vi "Create_Trajectory_Using_PathfinderSwerve_ORIG.vi"() -> ()   [LabVIEW 2019]
uses:
  <vilib>/Rock Robotics/WPI/ThirdParty/JAS_Junk/JaciPathFinderLib/VIs/Waypoint.ctl
  <vilib>/Rock Robotics/WPI/ThirdParty/JAS_Junk/TrajLib/TRAJ_STATE.ctl
  <vilib>/Rock Robotics/WPI/ThirdParty/JAS_Junk/TrajLib/POSE2D.ctl
  <vilib>/Rock Robotics/WPI/ThirdParty/JAS_Junk/TrajLib/TRANSLATION2D.ctl
  <vilib>/Rock Robotics/WPI/ThirdParty/JAS_Junk/TrajLib/ROTATION2D.ctl
  <vilib>/Rock Robotics/WPI/ThirdParty/JAS_Junk/TrajLib/UTIL_PATHFINDER_CONFIG.ctl
  <vilib>/Rock Robotics/WPI/ThirdParty/JAS_Junk/TrajLib/DISPLAY_WAYPOINT.ctl
  <vilib>/Rock Robotics/WPI/ThirdParty/JAS_Junk/JaciPathFinderLib/Pathfinder.lvlib
  <vilib>/Rock Robotics/WPI/ThirdParty/JAS_Junk/TrajLib/Trajectory_Library.lvlib
panel:
  in  "End Program":bool
  in  "Tab Control":T1(tab)
  in  "max_velocity":dbl=58.0
  in  "max_acceleration":dbl=65.0
  in  "max_jerk":dbl=70.0
  in  "wheelbase_width":dbl=20.866
  in  "Real max\n speed":dbl=65.0
  in  "wheelbase_depth":dbl=28.0
  in  "mode":u32(ring) items=["SWERVE_DEFAULT"]
  out "max speed":dbl
  out "Path \nSpeed > \nMax":bool
  out "Complete,\nReady to \nSave file":bool
  in  "Calculate\nPath":bool
  out "Path calculation error":errorcluster
  in  "sample_count":i32=100000
  in  "Path Results\ndT":dbl=0.02 format="%7.3f"
  in  "?":T2[](array[typedef])=[{"x"=15.0, "y"=105.0, "angle"=-45.0}, {"x"=105.0, "y"=65.0, "angle"=0.0}, {"x"=210.0, "y"=106.0, "angle"=45.0}]
  out "Position":cluster{dbl[], dbl[]}[](graph)
  out "Path Data":cluster{dbl[], dbl[]}[](graph)
  out "Traj States\nSize":i32
  out "Trajectory States":T3[](array[typedef]) {"POSE"."ROTATION"."SIN" format="%13.4f"; "POSE"."ROTATION"."COS" format="%13.4f"; "POSE"."ROTATION"."VALUE" format="%13.4f"; "POSE"."TRANSLATION"."Y" format="%14.3f"; "POSE"."TRANSLATION"."X" format="%14.3f"}
  out "File Saved\nWithout\nError":bool
  in  "Trajectory Type":enum32{"Radio Selection 1", "Radio Selection 2"}(radio)
  out "File Creation\nError":errorcluster
  in  "Trajectory File Comment":string
  in  "Trajectory File Name":path
  in  "CreateCmdList":bool
  # "Create trajectory using \"Jaci's Pathfinder\"  (Display for swerve drive robot)"
  # "Instructions:\n----------------  \nThis utility will create a trajectory,, show the data on the various tabs, and optionally write a \"robot relative\" trajectory to a \nfile. To use this utility:\n\n1) Read all of these instructions!\n2) Define the Robot Data. on the \"Robot Data\" tab.\n3) Define the \"Path Definition\" on the \"Define / Create Trajectory\" tab.  These are the beginning and ending positions/headings, and \n     internal positions/headings.\n4) Define the time increment.  0.020 is chosen since that matches the normal robot loop time.\n5) Define \"sample count\".  This is an internal PathFinder variable.  Leaving the value as default should work correctly.  Making \n    the value a little smaller will speed the program up a little.\n6) Press the \"Calculate Path\".  If a good path was calculated it will be displayed on the \"Field Position tab, and the \"Complete, \n    Ready to Save\" indicator will light.  The path can be recalculated many times before performing any other action.\n\nAfter a Path has been calculated, the \"trajectory can be written to a file.  The absolute path is converted to a robot relative \ntrajectory.  To do this:\n1) Enter a comment to be included in the file.  Anything can be entered.\n2) Select the file name.\n3) Select the type of trajectory to save, absolute or relative.\n4) Press \"Create Trajectory File\"  If an error occurs it will be displayed in the File Creation Error indicator.\n\nNotes:\n---------\n- All the robot parameters, path, and field dimensions are in INCHES, and DEGREES.  The resulting trajectory is converted to \n   METERS, and RADIANS to match the rest of this library!\n- The pathfinder path generation logic doesn't account distribution of speed to the left and right wheels.  As a result the \n   maximum speed can be exceeded.If this happens, but Path Speed > Max light will light and Ready to Execute will not \n   light.  Lower the maximum speed in the Robot Data tab and recalulate the path.  (CURRENTLY THIS LOGIC IS NOT COMPLETE.)\n- 2019 playing field size - width: 26 ft 11.25 In = 323.25 in , length: 52 ft 5.25 in = 629.25 in  (I didn't verify this for the 2020 version.)"
  # "ROBOT DATA"
  # "INCHES/SEC"
  # "INCHES/SEC"
  # "INCHES/SEC^2"
  # "INCHES/SEC^3"
  # "Simulated robot wheelbase is: 20.866"
  # "INCHES"
  # "Simulated robot max speed is: 68.266"
  # "INCHES"
  # "PATH DEFINITION"
  # "SEC"
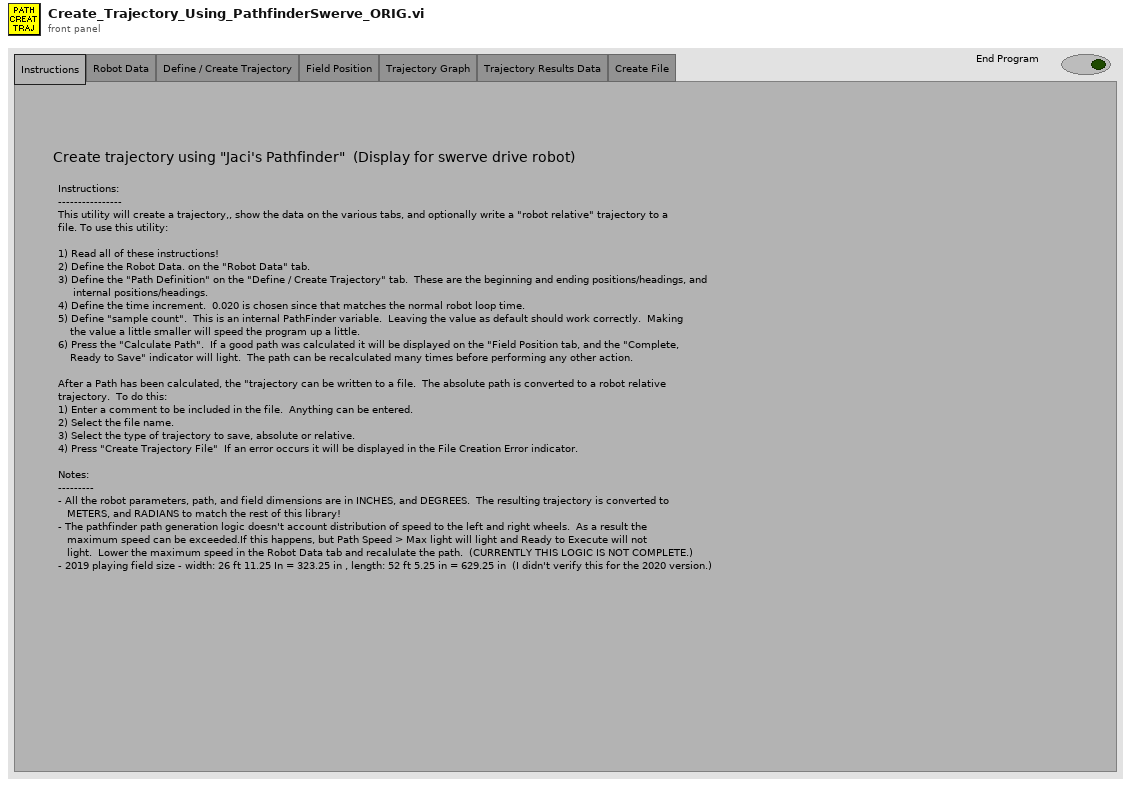
[diagram p1: front panel]
types:
  T1 = enum32{"Instructions", "Robot Data", "Define / Create Trajectory", "Field Position", "Trajectory Graph", "Trajectory Results Data", "Create File"}
  T2 = typedef "Pathfinder.lvlib/Waypoint.ctl" = cluster{"x":dbl, "y":dbl, "angle":dbl}
  T3 = typedef "Trajectory_Library.lvlib/TRAJ_STATE.ctl" = cluster{"TimeSeconds":dbl, "Velocity":dbl, "Acceleration":dbl, "POSE":T4, "Curvature":dbl}
  T4 = typedef "Trajectory_Library.lvlib/POSE2D.ctl" = cluster{"TRANSLATION":T5, "ROTATION":T6}
  T5 = typedef "Trajectory_Library.lvlib/TRANSLATION2D.ctl" = cluster{"X":dbl, "Y":dbl}
  T6 = typedef "Trajectory_Library.lvlib/ROTATION2D.ctl" = cluster{"VALUE":dbl, "COS":dbl, "SIN":dbl}
  T7 = typedef "Trajectory_Library.lvlib/DISPLAY_WAYPOINT.ctl" = cluster{"X":dbl, "Y":dbl, "ANGLE":dbl}
  T8 = typedef "Trajectory_Library.lvlib/UTIL_PATHFINDER_CONFIG.ctl" = cluster{"PathfinderType - 0 tank 1 serve":i32, "PathMaxVelocity - inches per sec":dbl, "MaxAcceleration - inches per sec2":dbl, "MaxJerk--Inches per sec2":dbl, "TimeDelta-Seconds":dbl, "SampleCount":i32, "WheelbaseWidth-inches":dbl, "WheelbaseDepth-inches":dbl, "SwerveType":i32, "ActualMaxVelocity-inches per sec":dbl}
  T9 = typedef "Trajectory_Library.lvlib/TRAJECTORY.ctl" = cluster{"TotalTImeSecs":dbl, "States":T3[]}
  T10 = typedef "Pathfinder.lvlib/Segment.ctl" = cluster{"dt":dbl, "x":dbl, "y":dbl, "position":dbl, "velocity":dbl, "acceleration":dbl, "jerk":dbl, "heading":dbl}
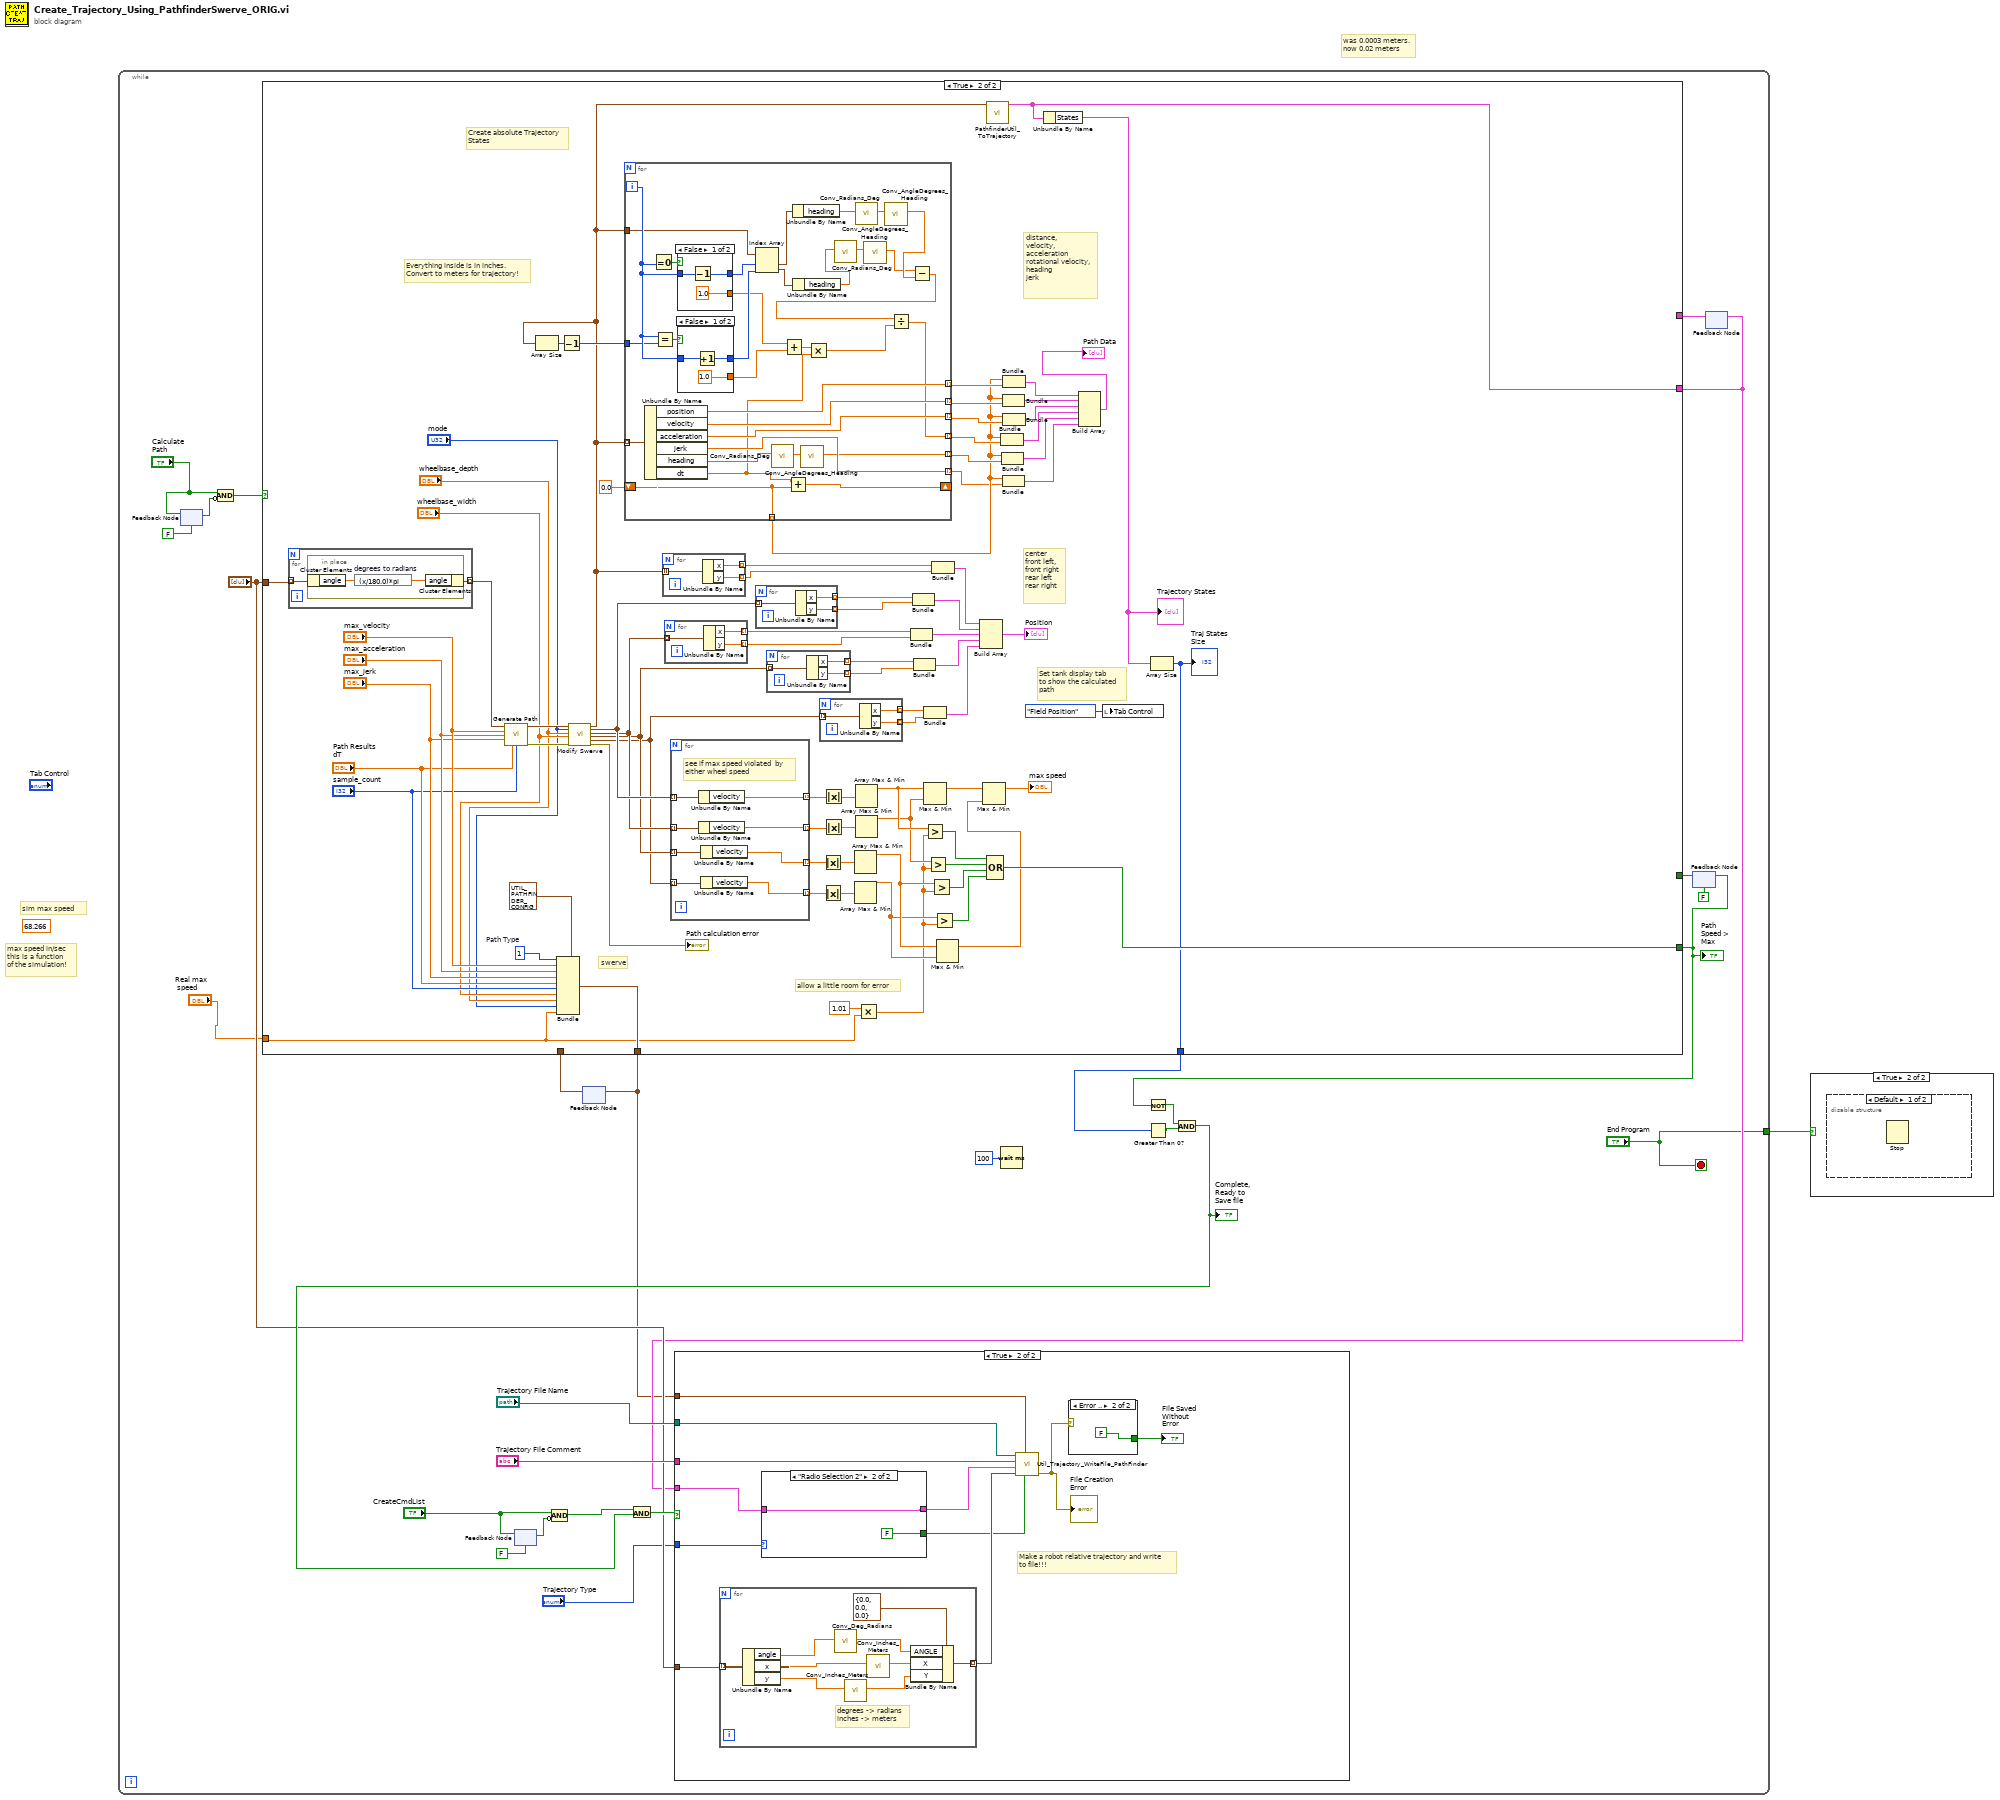
[diagram p0: block diagram]
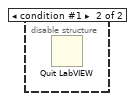
[diagram p3: hidden frame]
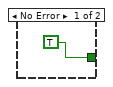
[diagram p5: hidden frame]
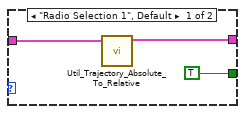
[diagram p6: hidden frame]
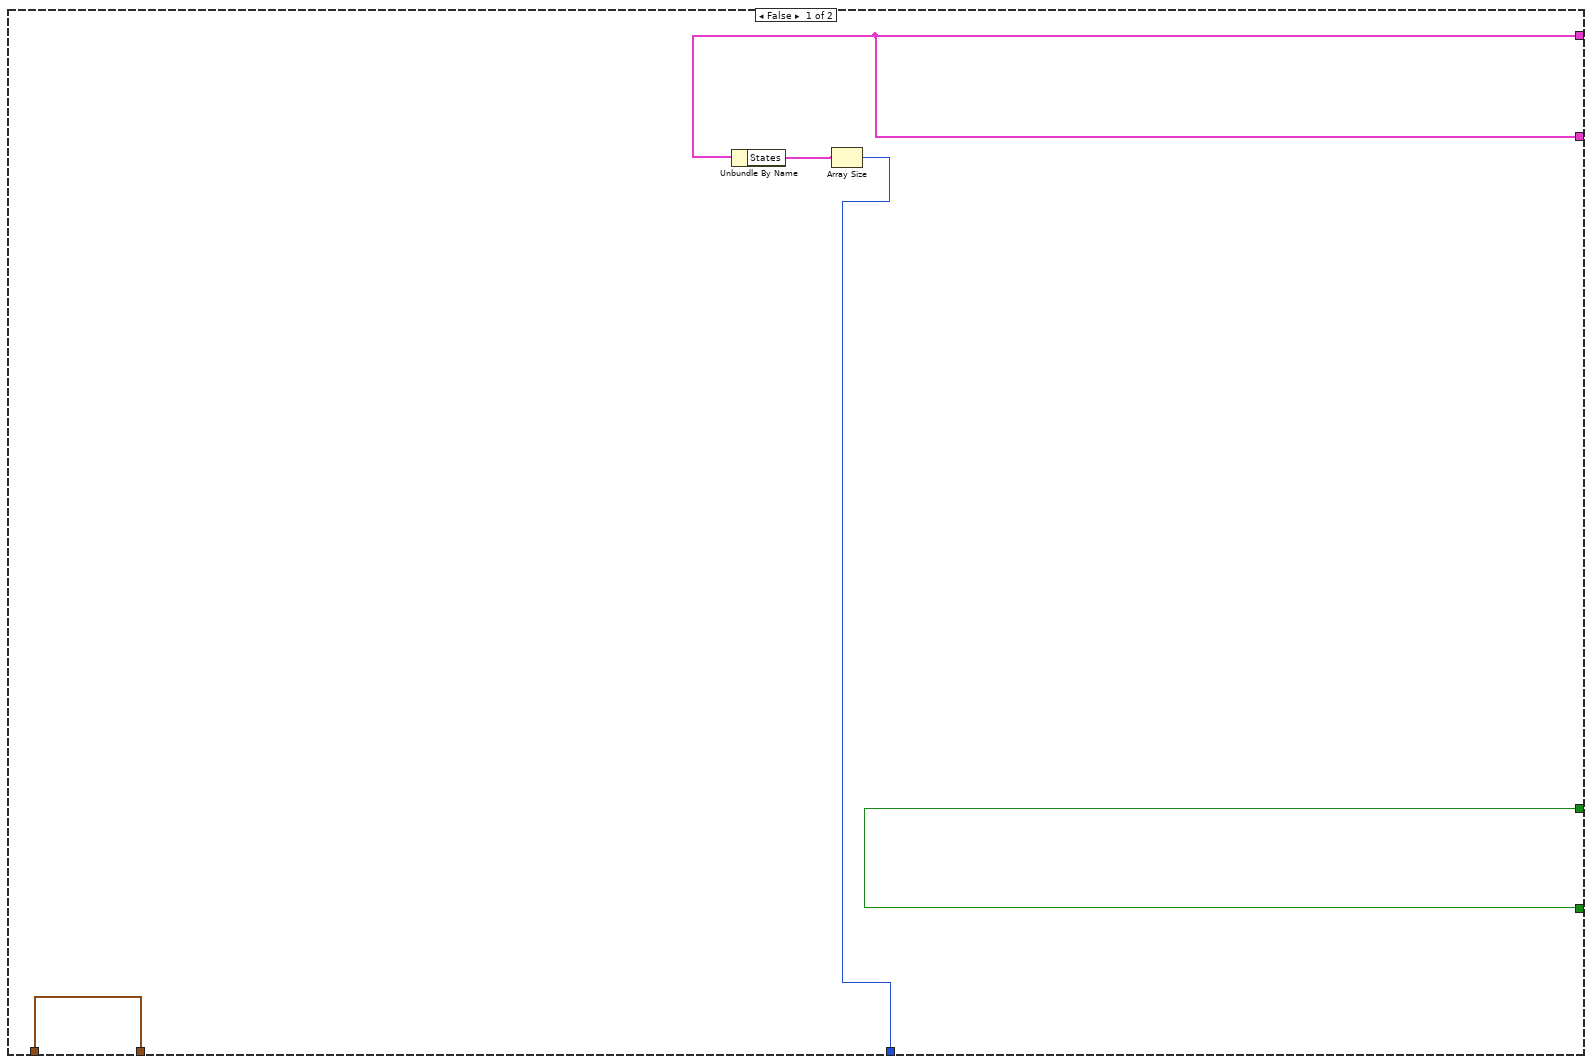
[diagram p7: hidden frame]
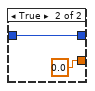
[diagram p8: hidden frame]
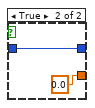
[diagram p9: hidden frame]
diagram:
  (unwired) 68.266 ("x")
  # "was 0.0003 meters.\nnow 0.02 meters"
  # "sim max speed"
  # "max speed in/sec\nthis is a function\nof the simulation!"
  n1 = while {
    tunnel: ["End Program"] -> w1
    stop <- "End Program" stop-if-true
    n2 = feedback #1(FALSE ("CreateCmdList")) -> (w10:bool)
    n3 = feedback-in #1("Calculate\nPath") -> ()
    n4 = Compound Arithmetic op=AND("Calculate\nPath", invert w10) -> (w7:bool)
    n5 = feedback-in #2("CreateCmdList") -> ()
    n6 = feedback #2(FALSE ("CreateCmdList")) -> (w13:bool)
    n7 = Compound Arithmetic op=AND("CreateCmdList", invert w13) -> (w12:bool)
    n8 = feedback #3() -> (w2:T8)  [unwired: 1 in]
    n9 = Wait (ms)(milliseconds to wait=u32 100) -> ()  [unwired: 1 out]
    n10 = feedback #4(FALSE) -> (w26:bool)
    n11 = feedback #5() -> (w22:T9)  [unwired: 1 in]
    n12 = case shown="True" w7 {
      tunnel: "Real max\n speed" -> [_ w62]
      tunnel: [w60 w127] -> w23
      tunnel: w26 -> [w60 _]
      tunnel: "?" -> [_ w126]
      tunnel: [w57 w106] -> w16
      tunnel: w22 -> [w57 _]
      tunnel: [w59 w120] -> w15
      tunnel: [w56 w65] -> w3
      tunnel: w2 -> [w56 _]
      frame False {
        n13 = Unbundle By Name(w57) -> ("States"=w58:T3[])
        n14 = Array Size(array=w58) -> (size(s)=w59:i32)
      }
      frame True {
        w74 = 1  # Path Type
        # "allow a little room for error"
        # "center\nfront left,\nfront right\nrear left\nrear right"
        # "distance,\nvelocity,\nacceleration\nrotational velocity,\nheading\njerk"
        # "swerve"
        # "Everything inside is in inches.\nConvert to meters for trajectory!"
        # "Create absolute Trajectory\nStates"
        # "Set tank display tab\nto show the calculated\npath"
        n15 = for {
          tunnel: w126 -> [w157] mode=indexing
          tunnel: [w156] -> w139 mode=indexing
          n16 = in-place {
            n17 = in-place-cluster #6(w157) -> ("angle"=w159:dbl)
            n18 = expression code="(x/180.0)*pi" "degrees to radians"(w159) -> (w158:dbl)
            n19 = in-place-cluster #6("angle"=w158) -> (w156:T2)
          }
        }
        n20 = call <vilib>:"Generate Path.vi"("path"=w139, "max_velocity"="max_velocity", "max_acceleration"="max_acceleration", "max_jerk"="max_jerk", "dt (.001)"="Path Results\ndT", "sample_count (100000)"="sample_count") -> ("Segments"=w140:T10[], "error out"=w96:errorcluster)  [unwired: 8 in]
        n21 = Bundle(cluster=T8 {"PathfinderType - 0 tank 1 serve"=0, "PathMaxVelocity - inches per sec"=0.0, "MaxAcceleration - inches per sec2"=0.0, "MaxJerk--Inches per sec2"=0.0, "TimeDelta-Seconds"=0.0, "SampleCount"=0, "WheelbaseWidth-inches"=0.0, "WheelbaseDepth-inches"=0.0, "SwerveType"=0, "ActualMaxVelocity-inches per sec"=0.0} ("UTIL_PATHFINDER_CONFIG"), "PathfinderType - 0 tank 1 serve"=w74, "PathMaxVelocity - inches per sec"="max_velocity", "MaxAcceleration - inches per sec2"="max_acceleration", "MaxJerk--Inches per sec2"="max_jerk", "TimeDelta-Seconds"="Path Results\ndT", "SampleCount"="sample_count", "WheelbaseWidth-inches"="wheelbase_width", "WheelbaseDepth-inches"="wheelbase_depth", "SwerveType"="mode", "ActualMaxVelocity-inches per sec"=w62) -> (w65:T8)
        n22 = call <vilib>:"Modify Swerve.vi"("Original"=w140, "mode"="mode", "wheelbase_depth"="wheelbase_depth", "wheelbase_width"="wheelbase_width", "error in"=w96) -> ("Original"=w97:T10[], "front_left out"=w80:T10[], "front_right out"=w79:T10[], "back_left out"=w78:T10[], "back_right out"=w77:T10[], "error out"=→"Path calculation error":errorcluster)  [unwired: 9 in]
        n23 = Array Size(array=w97) -> (size(s)=w99:i32)
        n24 = Decrement(x=w99) -> (x-1=w98:i32)
        n25 = for {
          tunnel: w97 -> [w200] mode=indexing
          shift-right: [w198] -> _
          shift-left: 0.0 -> [w199]
          tunnel: [w199] -> w102 mode=indexing
          tunnel: [w191] -> w103 mode=indexing
          tunnel: [w197] -> w101 mode=indexing
          tunnel: [w196] -> w111 mode=indexing
          tunnel: [w195] -> w110 mode=indexing
          tunnel: [w194] -> w105 mode=indexing
          tunnel: [w177] -> w104 mode=indexing
          tunnel: w97 -> [w183]
          tunnel: w98 -> [w176]
          i -> [w188]
          n26 = Unbundle By Name(w200) -> ("position"=w194:dbl, "velocity"=w195:dbl, "acceleration"=w196:dbl, "jerk"=w197:dbl, "heading"=w193:dbl, "dt"=w179:dbl)
          n27 = Equal To 0?(x=w188) -> (x = 0?=w190:bool)
          n28 = Equal?(x=w188, y=w176) -> (x = y?=w189:bool)
          n29 = case shown="False" w190 {
            tunnel: w188 -> [w208 w209]
            tunnel: [1.0 0.0] -> w180
            tunnel: [w206 w209] -> w185
            frame False {
              n30 = Decrement(x=w208) -> (x-1=w206:i32)
            }
            frame True {
            }
          }
          n31 = case shown="False" w189 {
            tunnel: [1.0 0.0] -> w181
            tunnel: w188 -> [w202 w204]
            tunnel: [w201 w204] -> w184
            frame False {
              n32 = Increment(x=w202) -> (x+1=w201:i32)
            }
            frame True {
            }
          }
          n33 = Index Array(array=w183, index #1=w185, index #2=w184) -> (element #1=w187:T10, element #2=w186:T10)
          n34 = call <vilib>:"Conv_Radians_Deg.vi"("Radians"=w193) -> ("Degrees"=w192:dbl)  [unwired: 10 in]
          n35 = Add(x=w180, y=w181) -> (x+y=w182:dbl)
          n36 = Add(x=w179, y=w199) -> (x+y=w198:dbl)
          n37 = Unbundle By Name(w187) -> ("heading"=w173:dbl)
          n38 = Unbundle By Name(w186) -> ("heading"=w171:dbl)
          n39 = call <vilib>:"Conv_AngleDegrees_Heading.vi"("Degrees"=w192) -> ("Heading Degrees"=w191:dbl)  [unwired: 10 in]
          n40 = Multiply(x=w182, y=w179) -> (x*y=w178:dbl)
          n41 = call <vilib>:"Conv_Radians_Deg.vi"("Radians"=w171) -> ("Degrees"=w170:dbl)  [unwired: 10 in]
          n42 = call <vilib>:"Conv_Radians_Deg.vi"("Radians"=w173) -> ("Degrees"=w174:dbl)  [unwired: 10 in]
          n43 = call <vilib>:"Conv_AngleDegrees_Heading.vi"("Degrees"=w170) -> ("Heading Degrees"=w169:dbl)  [unwired: 10 in]
          n44 = call <vilib>:"Conv_AngleDegrees_Heading.vi"("Degrees"=w174) -> ("Heading Degrees"=w172:dbl)  [unwired: 10 in]
          n45 = Subtract(x=w169, y=w172) -> (x-y=w175:dbl)
          n46 = Divide(x=w175, y=w178) -> (x/y=w177:dbl)
        }
        n47 = for {
          tunnel: w97 -> [w162] mode=indexing
          tunnel: [w161] -> w136 mode=indexing
          tunnel: [w160] -> w137 mode=indexing
          n48 = Unbundle By Name(w162) -> ("x"=w161:dbl, "y"=w160:dbl)
        }
        n49 = for {
          tunnel: w79 -> [w165] mode=indexing
          tunnel: [w164] -> w132 mode=indexing
          tunnel: [w163] -> w133 mode=indexing
          n50 = Unbundle By Name(w165) -> ("x"=w164:dbl, "y"=w163:dbl)
        }
        n51 = for {
          tunnel: w80 -> [w155] mode=indexing
          tunnel: w79 -> [w154] mode=indexing
          tunnel: [w153] -> w125 mode=indexing
          tunnel: [w152] -> w123 mode=indexing
          tunnel: w77 -> [w151] mode=indexing
          tunnel: w78 -> [w150] mode=indexing
          tunnel: [w149] -> w93 mode=indexing
          tunnel: [w148] -> w92 mode=indexing
          # "see if max speed violated  by\neither wheel speed"
          n52 = Unbundle By Name(w155) -> ("velocity"=w153:dbl)
          n53 = Unbundle By Name(w154) -> ("velocity"=w152:dbl)
          n54 = Unbundle By Name(w150) -> ("velocity"=w149:dbl)
          n55 = Unbundle By Name(w151) -> ("velocity"=w148:dbl)
        }
        n56 = for {
          tunnel: w80 -> [w168] mode=indexing
          tunnel: [w167] -> w130 mode=indexing
          tunnel: [w166] -> w131 mode=indexing
          n57 = Unbundle By Name(w168) -> ("x"=w167:dbl, "y"=w166:dbl)
        }
        n58 = for {
          tunnel: w78 -> [w147] mode=indexing
          tunnel: [w146] -> w84 mode=indexing
          tunnel: [w145] -> w83 mode=indexing
          n59 = Unbundle By Name(w147) -> ("x"=w146:dbl, "y"=w145:dbl)
        }
        n60 = for {
          tunnel: w77 -> [w144] mode=indexing
          tunnel: [w143] -> w82 mode=indexing
          tunnel: [w142] -> w81 mode=indexing
          n61 = Unbundle By Name(w144) -> ("x"=w143:dbl, "y"=w142:dbl)
        }
        n62 = Absolute Value(x=w93) -> (abs(x)=w95:dbl[])
        n63 = Absolute Value(x=w92) -> (abs(x)=w94:dbl[])
        n64 = Absolute Value(x=w125) -> (abs(x)=w124:dbl[])
        n65 = Absolute Value(x=w123) -> (abs(x)=w122:dbl[])
        n66 = Array Max & Min(array=w95) -> (max value=w89:dbl)  [unwired: 3 out]
        n67 = Array Max & Min(array=w94) -> (max value=w88:dbl)  [unwired: 3 out]
        n68 = Array Max & Min(array=w124) -> (max value=w119:dbl)  [unwired: 3 out]
        n69 = Array Max & Min(array=w122) -> (max value=w118:dbl)  [unwired: 3 out]
        n70 = Multiply(x=1.01, y=w62) -> (x*y=w63:dbl)
        n71 = Bundle(w132, w133) -> (w134:cluster{dbl[], dbl[]})  [unwired: 1 in]
        n72 = Bundle(w130, w131) -> (w135:cluster{dbl[], dbl[]})  [unwired: 1 in]
        n73 = Bundle(w84, w83) -> (w76:cluster{dbl[], dbl[]})  [unwired: 1 in]
        n74 = Bundle(w82, w81) -> (w75:cluster{dbl[], dbl[]})  [unwired: 1 in]
        n75 = Max & Min(x=w119, y=w118) -> (max(x,y)=w86:dbl)  [unwired: 1 out]
        n76 = Greater?(x=w119, y=w63) -> (0:w128:bool)
        n77 = Greater?(x=w118, y=w63) -> (0:w121:bool)
        n78 = Greater?(x=w89, y=w63) -> (0:w91:bool)
        n79 = Bundle(w136, w137) -> (w138:cluster{dbl[], dbl[]})  [unwired: 1 in]
        n80 = Greater?(x=w88, y=w63) -> (0:w90:bool)
        n81 = Max & Min(x=w89, y=w88) -> (max(x,y)=w87:dbl)  [unwired: 1 out]
        n82 = Build Array(w138, w135, w134, w76, w75) -> (→"Position":cluster{dbl[], dbl[]}[])
        n83 = Max & Min(x=w86, y=w87) -> (max(x,y)=→"max speed":dbl)  [unwired: 1 out]
        n84 = call <vilib>:"PathfinderUtil_ToTrajectory.vi"("Pathfinder Path"=w97) -> ("TRAJECTORY"=w106:T9)  [unwired: 10 in]
        n85 = Compound Arithmetic op=OR(w128, w121, w91, w90) -> (w127:bool)
        n86 = Bundle(w102, w104) -> (w114:cluster{dbl[], dbl[]})  [unwired: 1 in]
        n87 = Bundle(w102, w103) -> (w113:cluster{dbl[], dbl[]})  [unwired: 1 in]
        n88 = Bundle(w102, w110) -> (w116:cluster{dbl[], dbl[]})  [unwired: 1 in]
        n89 = Bundle(w102, w101) -> (w100:cluster{dbl[], dbl[]})  [unwired: 1 in]
        n90 = Bundle(w102, w105) -> (w117:cluster{dbl[], dbl[]})  [unwired: 1 in]
        n91 = Bundle(w102, w111) -> (w115:cluster{dbl[], dbl[]})  [unwired: 1 in]
        n92 = Unbundle By Name(w106) -> ("States"=w108:T3[])
        "Trajectory States" <- w108
        n93 = Build Array(w117, w116, w115, w114, w113, w100) -> (→"Path Data":cluster{dbl[], dbl[]}[])
        n94 = local write "Tab Control"(T1."Field Position" ("Tab Control")) -> ()
        n95 = Array Size(array=w108) -> (size(s)=w120:i32)
        "Traj States\nSize" <- w120
      }
    }
    "Path \nSpeed > \nMax" <- w23
    n96 = feedback-in #3(w3) -> ()
    n97 = Not(x=w23) -> (.not. x?=w24:bool)
    n98 = Greater Than 0?(x=w15) -> (x > 0?=w25:bool)
    n99 = And(x=w24, y=w25) -> (x .and. y?=w18:bool)
    "Complete,\nReady to \nSave file" <- w18
    n100 = And(x=w12, y=w18) -> (x .and. y?=w19:bool)
    n101 = case shown="True" w19 {
      tunnel: "Trajectory File Name" -> [_ w39]
      tunnel: "Trajectory File Comment" -> [_ w38]
      tunnel: w16 -> [_ w34]
      tunnel: "?" -> [_ w37]
      tunnel: "Trajectory Type" -> [_ w33]
      tunnel: w3 -> [_ w29]
      frame False {
      }
      frame True {
        # "Make a robot relative trajectory and write\nto file!!!"
        n102 = for {
          tunnel: w37 -> [w55] mode=indexing
          tunnel: [w54] -> w36 mode=indexing
          # "degrees -> radians\ninches -> meters"
          n103 = Unbundle By Name(w55) -> ("angle"=w48:dbl, "x"=w53:dbl, "y"=w51:dbl)
          n104 = call <vilib>:"Conv_Deg_Radians.vi"("Degress"=w48) -> ("Radians"=w49:dbl)  [unwired: 10 in]
          n105 = call <vilib>:"Conv_Inches_Meters.vi"("INCH"=w51) -> ("Meters"=w50:dbl)  [unwired: 10 in]
          n106 = call <vilib>:"Conv_Inches_Meters.vi"("INCH"=w53) -> ("Meters"=w52:dbl)  [unwired: 10 in]
          n107 = Bundle By Name(cluster=T7 {"X"=0.0, "Y"=0.0, "ANGLE"=0.0} ("UTIL_WAYPOINT"), "ANGLE"=w49, "X"=w52, "Y"=w50) -> (w54:T7)
        }
        n108 = case shown="\"Radio Selection 2\"" w33 {
          tunnel: w34 -> [w44 w46]
          tunnel: [w43 w46] -> w35
          tunnel: [TRUE FALSE] -> w30
          frame "Radio Selection 1", Default {
            n109 = call <vilib>:"Util_Trajectory_Absolute_To_Relative.vi"("absTRAJECTORY"=w44) -> ("outputRelativeTRAJECTORY"=w43:T9)  [unwired: 10 in]
          }
          frame "Radio Selection 2" {
          }
        }
        n110 = call <vilib>:"Util_Trajectory_WriteFile_PathFinder.vi"("Trajectory Is Relative"=w30, "UTIL_PATHFINDER_CONFIG"=w29, "UtilityWayPoints"=w36, "TRAJECTORY"=w35, "Comment"=w38, "Trajectory File Name"=w39) -> ("error out"=w32:errorcluster)  [unwired: 5 in]
        "File Creation\nError" <- w32
        n111 = case shown="Error .." w32 {
          tunnel: [TRUE ("File Saved\nWithout\nError") FALSE ("File Saved\nWithout\nError")] -> w31
          frame No Error {
          }
          frame Error {
          }
        }
        "File Saved\nWithout\nError" <- w31
      }
    }
    n112 = feedback-in #4(w23) -> ()
    n113 = feedback-in #5(w16) -> ()
  }
  n114 = case shown="True" w1 {
    frame False {
    }
    frame True {
      n115 = disable-structure shown="Default" {
        frame condition #0 (active) {
          n116 = Stop() -> ()  [unwired: 1 in]
        }
        frame condition #1 {
          n117 = Quit LabVIEW() -> ()  [unwired: 1 in]
        }
      }
    }
  }
